vi "Print Report.vi"(0 "report in":refnum<class "NI_Excel.lvclass">, 5 "printer name (default)":string, 9 "number of copies (1)":i32=1, 11 "error in (no error)":errorcluster) -> (4 "report out":refnum<class "NI_Excel.lvclass">, 15 "error out":errorcluster)   [LabVIEW 2015, in "NI_Excel.lvclass"]
doc: "Prints a report to a designated printer or to the default printer on the computer."
uses:
  <vilib>/Utility/NIReport.llb/Excel/NI_Excel.lvclass
  <vilib>/Utility/NIReport.llb/Excel/NI_Excel.lvclass/NI_Excel.ctl
  <vilib>/addons/_office/NI_ReportGenerationToolkit.lvlib
  <vilib>/Utility/NIReport.llb/NI_ReportGenerationCore.lvlib
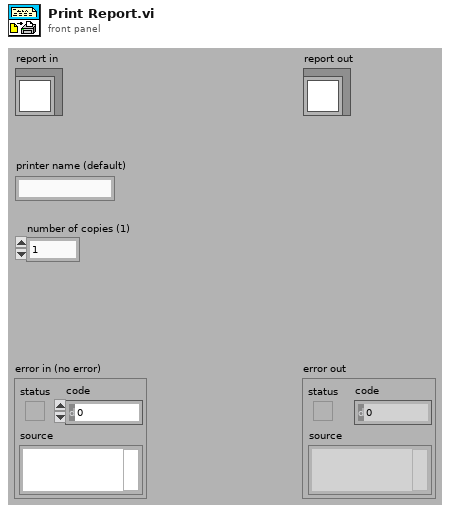
[diagram p1: front panel]
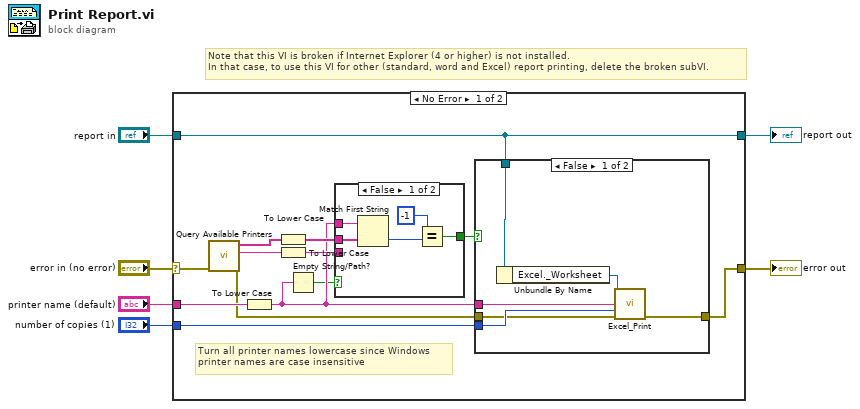
[diagram p0: block diagram]
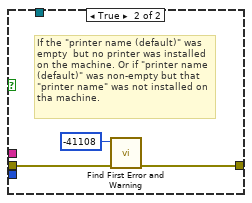
[diagram p2: hidden frame]
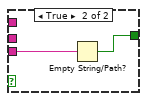
[diagram p3: hidden frame]
diagram:
  # "Note that this VI is broken if Internet Explorer (4 or higher) is not installed.\nIn that case, to use this VI for other (standard, word and Excel) report printing, delete the broken subVI."
  n1 = case shown="No Error" "error in (no error)" {
    selector: "error in (no error)" -> [w10 w37]
    tunnel: [w7 w37] -> w5
    tunnel: [w8 w36] -> w3
    tunnel: "report in" -> [w8 w36]
    tunnel: "printer name (default)" -> [w12 _]
    tunnel: "number of copies (1)" -> [w11 _]
    frame No Error {
      # "Turn all printer names lowercase since Windows\nprinter names are case insensitive"
      n2 = call <vilib>:"Query Available Printers.vi"("error in (no error)"=w10) -> ("error out"=w9:errorcluster, "default printer"=w16:string, "system configured printers"=w15:string[])  [unwired: 8 out]
      n3 = To Lower Case(string=w12) -> (all lower case string=w17:string)
      n4 = To Lower Case(string=w15) -> (all lower case string=w18:string[])
      n5 = To Lower Case(string=w16) -> (all lower case string=w19:string)
      n6 = Empty String/Path?(string/path=w17) -> (empty?=w13:bool)
      n7 = case shown="False" w13 {
        tunnel: w17 -> [w29 _]
        tunnel: [w30 w35] -> w14
        tunnel: w18 -> [w31 _]
        tunnel: w19 -> [_ w34]
        frame False {
          n8 = Match First String(2:w31, 3:w29) -> (0:w33:i32)  [unwired: 1 out]
          n9 = Equal?(x=-1 ("y"), y=w33) -> (x = y?=w30:bool)
        }
        frame True {
          n10 = Empty String/Path?(string/path=w34) -> (empty?=w35:bool)
        }
      }
      n11 = case shown="False" w14 {
        tunnel: w11 -> [w23 _]
        tunnel: w17 -> [w24 _]
        tunnel: w9 -> [w22 w27]
        tunnel: w8 -> [w21 _]
        tunnel: [w20 w26] -> w7
        frame False {
          n12 = Unbundle By Name(w21) -> ("Excel._Worksheet"=w25:refnum<k7>)
          n13 = call <vilib>:"Excel_Print.vi"("Excel._Worksheet"=w25, "printer name (default)"=w24, "number of copies (1)"=w23, "error in (no error)"=w22) -> ("error out"=w20:errorcluster)  [unwired: 11 out]
        }
        frame True {
          # "If the \"printer name (default)\" was empty  but no printer was installed on the machine. Or if \"printer name (default)\" was non-empty but that \"printer name\" was not installed on tha machine."
          n14 = call <vilib>:"Find First Error and Warning.vi"("error in (no error)"=w27, "error code"=-41108) -> ("error out"=w26:errorcluster)  [unwired: 5 out]
        }
      }
    }
    frame Error {
    }
  }
  "error out" <- w5
  "report out" <- w3
